vi "DPO_7K_Get_Channel_Position.vi"(8 "Error In":errorcluster, 10 "Channel":u16(ring) items=["Channel 1", "Channel 2", "Channel 3", "Channel 4", "Math 1", "Math 2", "Math 3", "Math 4", "Reference 1", "Reference 2", "Reference 3", "Reference 4"], 11 "VISA resource name in":refnum<visa-resource-name>) -> (0 "Error Out":errorcluster, 2 "Position":dbl, 3 "VISA resource name out":refnum<visa-resource-name>)   [LabVIEW 2020]
uses:
  subVI/Set_Configuration.ctl
  subVI/Return_To_Interface.ctl
panel:
  in  "Return to Interface":T1
  in  "Set":T2
  # "GET CHANNEL POSITION"
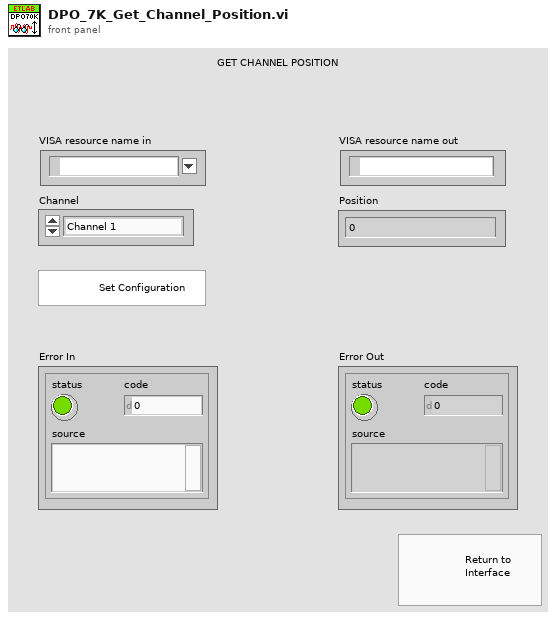
[diagram p1: front panel]
types:
  T1 = typedef "Return_To_Interface.ctl" = bool
  T2 = typedef "Set_Configuration.ctl" = bool
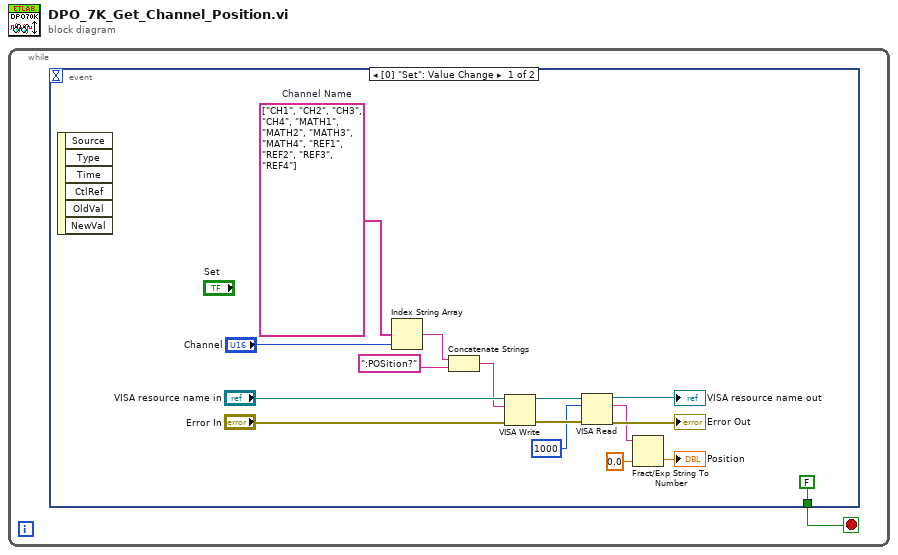
[diagram p0: block diagram]
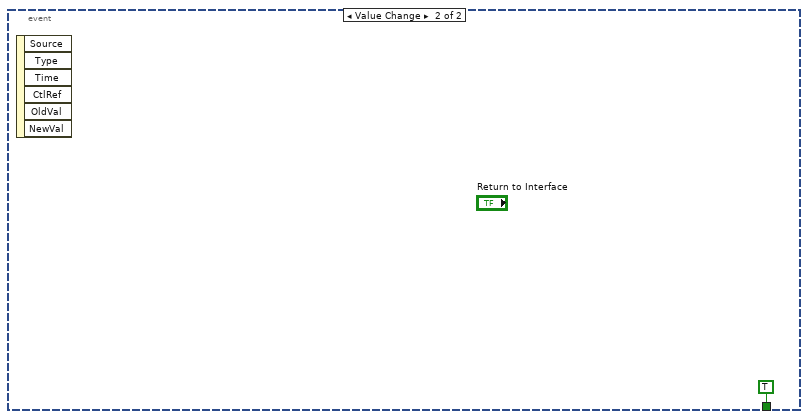
[diagram p2: hidden frame]
diagram:
  n1 = while {
    stop <- w1 stop-if-true
    n2 = event shown="[0] \"Set\": Value Change" {
      selector: _ -> [_ _]
      dyn-events: _ -> [_ _]
      timeout: _ -> [_ _]
      tunnel: [FALSE TRUE] -> w1
      event Value Change {
        w13 = string[] ["CH1", "CH2", "CH3", "CH4", "MATH1", "MATH2", "MATH3", "MATH4", "REF1", "REF2", "REF3", "REF4"]  # Channel Name
        n3 = event-data() -> ()  [unwired: 1 in, 6 out]
        n4 = Index String Array(1:"Channel", 2:w13) -> (0:w11:string)  [unwired: 1 in]
        n5 = Concatenate Strings(w11, ":POSition?" ("write buffer")) -> (w10:string)
        n6 = VISA Write(VISA resource name="VISA resource name in", write buffer=w10, error in (no error)="Error In") -> (VISA resource name out=w6:refnum<visa-resource-name>, error out=w7:errorcluster)  [unwired: 1 out]
        n7 = VISA Read(VISA resource name=w6, byte count=u32 1000, error in (no error)=w7) -> (VISA resource name out=→"VISA resource name out":refnum<visa-resource-name>, read buffer=w4:string, error out=→"Error Out":errorcluster)  [unwired: 1 out]
        n8 = Fract/Exp String To Number(string=w4, default (0 dbl)=0.0 ("default (0 DBL)")) -> (number=→"Position":dbl)  [unwired: 2 in, 1 out]
      }
      event Value Change {
        n9 = event-data() -> ()  [unwired: 1 in, 6 out]
      }
    }
  }
